vi "DEMO Updated UI State.vi"(8 "error in (no error)":errorcluster, 10 "State":T1) -> (0 "error out":errorcluster)   [LabVIEW 2020, in "StateMachine.lvlib"]
doc: "Broadcasts whenever the \"Update UI State\" private request was executed after a state change\n____\nHAMPEL SOFTWARE ENGINEERING v2.6.0 (2023-12-19 10:54)"
uses:
  StateMachine.lvlib
  HSE-SM/SM_States.ctl
  DEMO Updated UI State Argument--cluster.ctl
  HSE-SM/HSE-State-Machine.lvlib
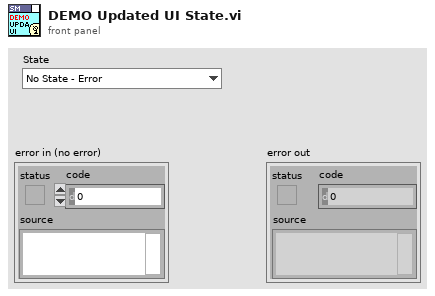
[diagram p1: front panel]
types:
  T1 = typedef "StateMachine.lvlib/HSE-State-Machine.lvlib/SM_States.ctl" = enum16{"No State - Error", "Error - Waiting For Action", "Initialising", "Standing by (idle)", "Waiting for External Trigger", "Polling for Signal Change", "Exiting"}
  T2 = typedef "StateMachine.lvlib/DEMO Updated UI State Argument--cluster.ctl" = cluster{"State":T1}
  T3 = typedef "StateMachine.lvlib/Broadcast Events--cluster.ctl" = cluster{"Module Did Init":refnum<user-event>, "Status Updated":refnum<user-event>, "Error Reported":refnum<user-event>, "Module Did Stop":refnum<user-event>, "Update Module Execution Status":refnum<user-event>, "System Message":refnum<user-event>, "DEMO Updated UI State":refnum<user-event>}
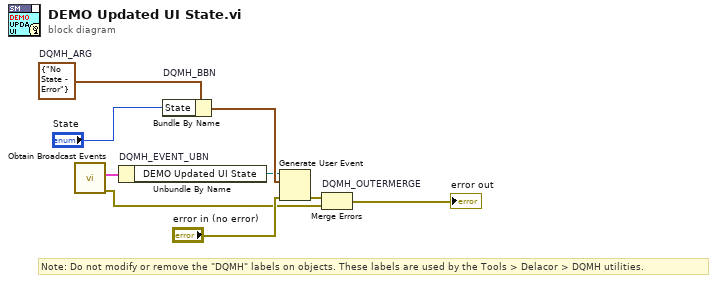
[diagram p0: block diagram]
diagram:
  w4 = T2 {"State"=enum."No State - Error"}  # DQMH_ARG
  # "Note: Do not modify or remove the \"DQMH\" labels on objects. These labels are used by the Tools > Delacor > DQMH utilities."
  n1 = call "Obtain Broadcast Events.vi"() -> ("error out"=w2:errorcluster, "StateMachine Broadcast Events"=w1:T3)  [unwired: 10 in]
  n2 = Unbundle By Name "DQMH_EVENT_UBN"(w1) -> ("DEMO Updated UI State"=w6:refnum<user-event>)
  n3 = Bundle By Name "DQMH_BBN"(cluster=w4, "State"="State") -> (w7:T2)
  n4 = Generate User Event(user event=w6, event data cluster=w7, error in="error in (no error)") -> (error out=w5:errorcluster)  [unwired: 1 in, 1 out]
  n5 = Merge Errors "DQMH_OUTERMERGE"(w5, w2) -> (→"error out":errorcluster)
